vi "1.5.5-Multiply.vi"(2 "Input A":fxp<+/-,18,1>, 3 "Input B":fxp<+/-,18,1>, 4 "Unique 8b identifier":u8) -> (1 "Timed out":bool, 7 "Output":fxp<+/-,18,1>)   [LabVIEW 2010]
doc: "Major note from gray:\nThere is a possibility that this vi will frack your shit. It is designed to be non re-entrant (clone copy), and it is also designed to support 2^8 clients, each client basically using the multiplication server periodically (and maintaining a unique 8b identifier). IF the server is monopolized by one client, this client may get screwed up by an identical looking but much older packet. The client's clone of this vi will maintain an 8 bit register to indicate a count but only 6 bits are read! 2^6 is 64 so, given the 69 memory locations the vi might be reading, there is a chance that it will read an incorect value (the 64th oldest one) from those five insecure locations. The timing of this vi is designed to maximize the chance that the first newest number is read, but it is possible that the channel watcher vi will execute before the value is added, and in this case the channel watcher will search through all 69 locations before searching the most likely one again. If this happens the watcher will notice this older datapoint in one of these 5 insecure locations and will use it instead of the new multiplication. \nThe solution to this problem is to avoid monopolizing channels and in the worst case divide the multiplication from one client between two clones."
uses:
  1.0-Hindbrain Global.vi
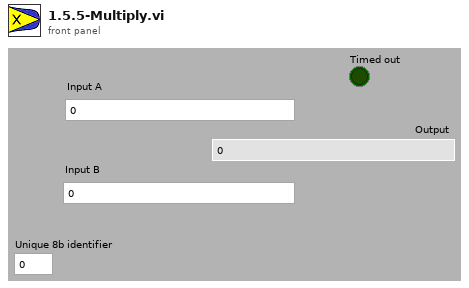
[diagram p1: front panel]
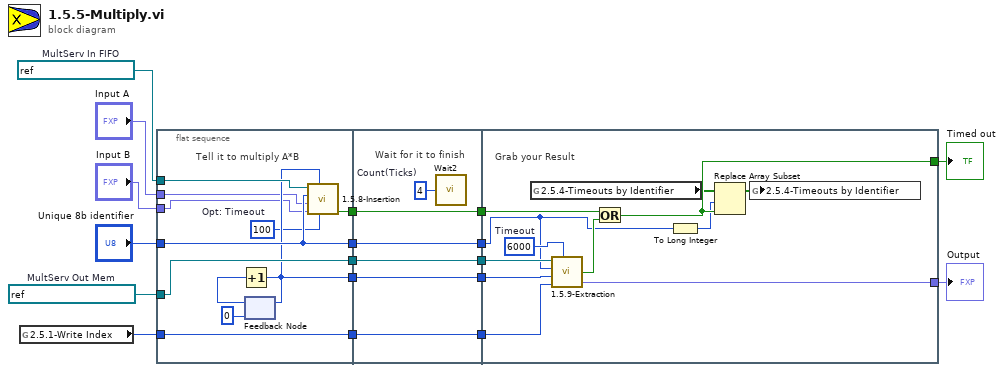
[diagram p0: block diagram]
diagram:
  w5 = refnum<k21> "1.5.3-MultServ In"  # MultServ In FIFO
  w6 = refnum<k21> "1.5.2-MultServ Out"  # MultServ Out Mem
  n1 = global read "1.0-Hindbrain Global.vi" "2.5.1-Write Index"() -> (w1:u32)
  n2 = flat-sequence {
    tunnel: [w29] -> w14
    tunnel: [w28] -> w13
    tunnel: [w25] -> w12
    tunnel: [w26] -> w11
    tunnel: "Unique 8b identifier" -> [w29]
    tunnel: w5 -> [w27]
    tunnel: w6 -> [w28]
    tunnel: w1 -> [w25]
    tunnel: "Input A" -> [w24]
    tunnel: "Input B" -> [w23]
    tunnel: [w19] -> w3
    tunnel: w14 -> [w35]
    tunnel: [w35] -> w10
    tunnel: w13 -> [w34]
    tunnel: [w34] -> w9
    tunnel: w12 -> [w33]
    tunnel: [w33] -> w8
    tunnel: w11 -> [w32]
    tunnel: [w32] -> w7
    tunnel: [w30] -> w4
    tunnel: w3 -> [w30]
    tunnel: w10 -> [w40]
    tunnel: w9 -> [w47]
    tunnel: w8 -> [w46]
    tunnel: w7 -> [w45]
    tunnel: [w44] -> w16
    tunnel: w4 -> [w41]
    tunnel: [w39] -> w2
    frame #0 {
      w20 = u8 100  # Opt: Timeout
      # "Tell it to multiply A*B"
      n3 = feedback #1(u8 0) -> (w22:u8)
      n4 = Increment(x=w22) -> (x+1=w26:u8)
      n5 = feedback-in #1(w26) -> ()
      n6 = call "1.5.8-Insertion.vi"("Opt: Timeout"=w20, "Counter Descriminator"=w26, "Input B"=w23, "Input A"=w24, "Channel Identifier"=w29, "FIFO"=w27) -> ("Timeout"=w19:bool)  [unwired: 5 in]
    }
    frame #1 {
      w31 = u32 4  # Count(Ticks)
      # "Wait for it to finish"
      n7 = call "Wait2"("Count(Ticks)"=w31) -> ()  [unwired: 1 out]
    }
    frame #2 {
      w42 = 6000  # Timeout
      # "Grab your Result"
      n8 = global read "1.0-Hindbrain Global.vi" "2.5.4-Timeouts by Identifier"() -> (w36:bool[])
      n9 = call "1.5.9-Extraction.vi"("Block Memory"=w47, "Watched Channel"=w40, "Count to match"=w45, "Writing Index Start"=w46, "Timeout"=w42) -> ("Timed out"=w43:bool, "Multiplication Result"=w44:fxp<+/-,18,1>)  [unwired: 1 out]
      n10 = Or(x=w41, y=w43) -> (x .or. y?=w39:bool)
      n11 = To Long Integer(number=w40) -> (32bit integer=w38:i32)
      n12 = Replace Array Subset(array=w36, new element=w39, index=w38) -> (w37:bool[])
      n13 = global write "1.0-Hindbrain Global.vi" "2.5.4-Timeouts by Identifier"(w37) -> ()
    }
  }
  "Output" <- w16
  "Timed out" <- w2
